vi "Parse Washer Debug Log.vi"(10 "Good Responses":cluster{"Bytes Data":u8[]}[](array[cluster])) -> (2 "Debug Log":string)   [LabVIEW 2011]
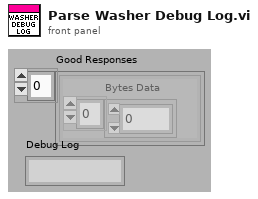
[diagram p1: front panel]
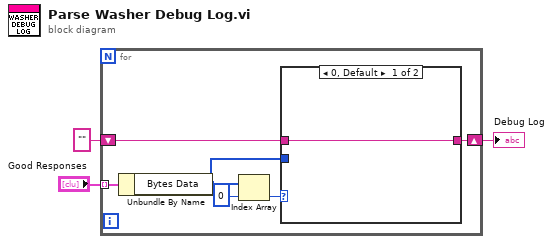
[diagram p0: block diagram]
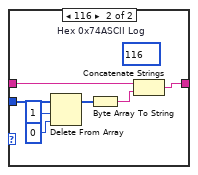
[diagram p2: hidden frame]
diagram:
  n1 = for {
    tunnel: "Good Responses" -> [w9] mode=indexing
    shift-right: [w5] -> w1
    shift-left: "" -> [w4]
    n2 = Unbundle By Name(w9) -> ("Bytes Data"=w6:u8[])
    n3 = Index Array(array=w6, index=0) -> (element=w7:u8)
    n4 = case shown="0, Default" w7 {
      tunnel: w6 -> [_ w14]
      tunnel: [w10 w12] -> w5
      tunnel: w4 -> [w10 w11]
      frame 0, Default {
      }
      frame 116 {
        (unwired) 116  # Hex 0x74ASCII Log
        n5 = Delete From Array(array=w14, length=1, index=0) -> (array with subset deleted=w17:u8[])  [unwired: 1 out]
        n6 = Byte Array To String(unsigned byte array=w17) -> (string=w13:string)
        n7 = Concatenate Strings(w11, w13) -> (w12:string)
      }
    }
  }
  "Debug Log" <- w1
